vi "Read Old GoTo Params.vi"(8 "error in (no error)":errorcluster, 11 "Parameters in":refnum<class "Parameters.lvclass">) -> (0 "error out":errorcluster, 2 "Old GoTo Params":T1={"PID gains Angle GoTo"={"(Kc)"=3.0, "(Ki)"=0.0, "(Kd)"=2.0}, "PID gains XY GoTo"={"(Kc)"=3.0, "(Ki)"=0.0, "(Kd)"=2.0}, "Max Params GoTo"={"Max output XY"=3.0, "MaxOutput Angle"=0.0}}, 3 "Parameters out":refnum<class "Parameters.lvclass">)   [LabVIEW 2020, in "Parameters.lvclass"]
uses:
  Parameters.lvclass
  Parameters.lvclass/Parameters.ctl
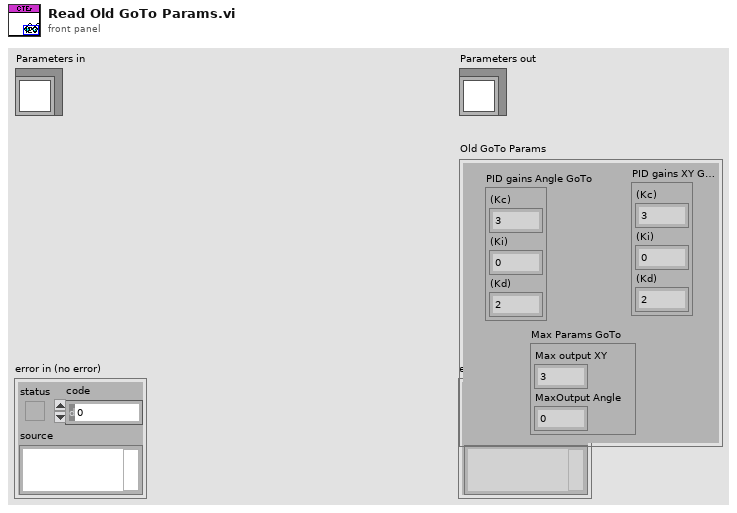
[diagram p1: front panel]
types:
  T1 = cluster{"PID gains Angle GoTo":cluster{"(Kc)":dbl, "(Ki)":dbl, "(Kd)":dbl}, "PID gains XY GoTo":cluster{"(Kc)":dbl, "(Ki)":dbl, "(Kd)":dbl}, "Max Params GoTo":cluster{"Max output XY":dbl, "MaxOutput Angle":dbl}}
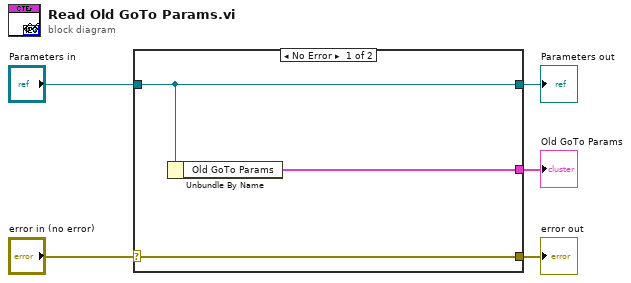
[diagram p0: block diagram]
diagram:
  n1 = case shown="No Error" "error in (no error)" {
    selector: "error in (no error)" -> [w8 w9]
    tunnel: [w8 w9] -> w4
    tunnel: [w7 w10] -> w2
    tunnel: "Parameters in" -> [w7 w10]
    tunnel: [w6 _] -> w1
    frame No Error {
      n2 = Unbundle By Name(w7) -> ("Old GoTo Params"=w6:T1)
    }
    frame Error {
    }
  }
  "error out" <- w4
  "Parameters out" <- w2
  "Old GoTo Params" <- w1
